vi "ZipUpCode.vi"() -> ()   [LabVIEW 2022 SP3]
uses:
  ViolinSubs/Mic/Mic_Global.vi
panel:
  out "error out":errorcluster
  out "Warnings":string
  out "Generated Zip File":path
  # "STEPS TO BUILD INSTALLERS\n\nZipUpCode first\n\nMac\n1. Build standalone - \n2. click on explore and compress the App folder\n2. drag it into the google drive\n\nPC \n0. grab zip file on the PC side - unzip\n1. open up Curtin1 in LabVIEW\n2. recompile and save all changes\n3. Build App\n4. build installer\n5. Zip up installer - and give it a name like ObieApp1_0b76\n6. copy that zip over to GoogleDrive:CurtinViolin:Code:PC"
  # "USE THE PC in the SHOP"
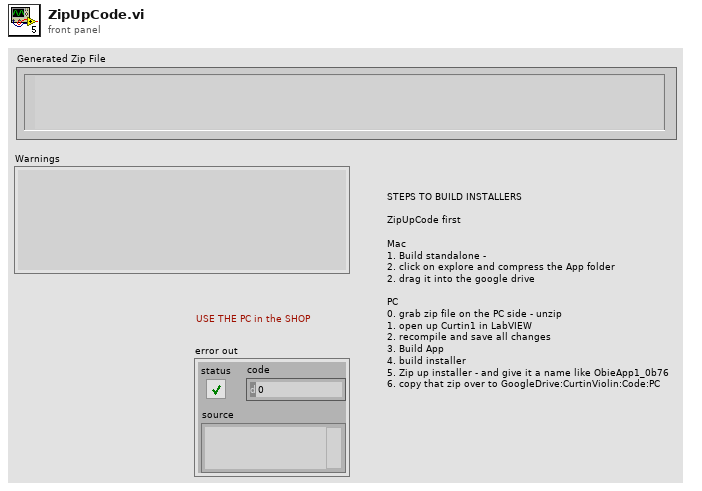
[diagram p1: front panel]
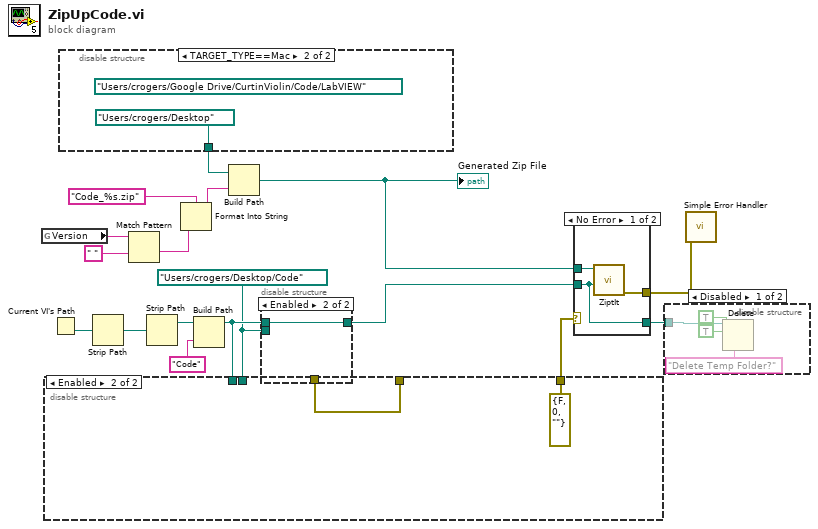
[diagram p0: block diagram]
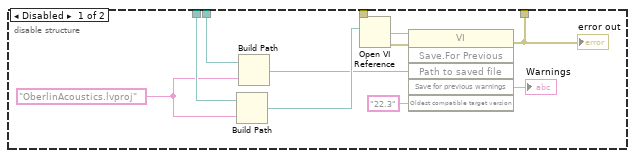
[diagram p3: hidden frame]
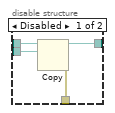
[diagram p4: hidden frame]
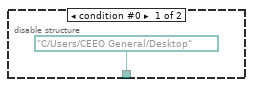
[diagram p6: hidden frame]
diagram:
  w1 = path "/Users/crogers/Desktop/Code"
  n1 = global read "Mic_Global.vi" "Version"() -> (w9:string)
  n2 = Current VI's Path() -> (path=w13:path)
  n3 = disable-structure shown="TARGET_TYPE==Mac" {
    disable-tunnel: [path "C:/Users/CEEO General/Desktop" ("default name") path "/Users/crogers/Desktop"] -> w18
    frame condition #0 {
    }
    frame condition #1 (active) {
      (unwired) path "/Users/crogers/Google Drive/CurtinViolin/Code/LabVIEW"
    }
  }
  n4 = Strip Path(path=w13) -> (stripped path=w12:path)  [unwired: 1 out]
  n5 = Match Pattern(string=w9, regular expression=" ") -> (after substring=w15:string)  [unwired: 1 in, 3 out]
  n6 = Strip Path(path=w12) -> (stripped path=w11:path)  [unwired: 1 out]
  n7 = Format Into String(format string="Code_%s.zip", w15) -> (resulting string=w14:string)  [unwired: 2 in, 1 out]
  n8 = Build Path(base path=w11, name or relative path="Code") -> (appended path=w2:path)
  n9 = Build Path(base path=w18, name or relative path=w14) -> (appended path=w8:path)
  "Generated Zip File" <- w8
  n10 = disable-structure shown="Enabled" {
    disable-tunnel: [w24 w25] -> w7
    disable-tunnel: w1 -> [w23 _]
    disable-tunnel: [w22 _] -> w6
    disable-tunnel: w2 -> [w21 w25]
    frame Disabled {
      n11 = Copy(10:w23, 11:w21) -> (0:w22:errorcluster, 3:w24:path)  [unwired: 3 in, 1 out]
    }
    frame Enabled {
    }
  }
  n12 = disable-structure shown="Enabled" {
    disable-tunnel: w6 -> [w32 _]
    disable-tunnel: [w30 errorcluster {"status"=FALSE, "code"=0, "source"=""} ("error out")] -> w5
    disable-tunnel: w2 -> [w29 _]
    disable-tunnel: w1 -> [w28 _]
    frame Disabled {
      w27 = "OberlinAcoustics.lvproj"
      n13 = Build Path(base path=w29, name or relative path=w27) -> (appended path=w35:path)
      n14 = Build Path(base path=w28, name or relative path=w27) -> (appended path=w26:path)
      n15 = Open VI Reference(vi path=w35, error in (no error)=w32) -> (vi reference=w36:refnum<vi>, error out=w31:errorcluster)  [unwired: 4 in]
      n16 = invoke class="VI" method="Save.For Previous"(reference=w36, error in=w31, "Path to saved file"=w26, "Oldest compatible target version"="22.3" ("Target Version")) -> (error out=w30:errorcluster, "Save for previous warnings"=→"Warnings":string)  [unwired: 2 in, 4 out]
      "error out" <- w30
    }
    frame Enabled {
    }
  }
  n17 = case shown="No Error" w5 {
    selector: w5 -> [_ w42]
    tunnel: w8 -> [w40 _]
    tunnel: w7 -> [w38 w41]
    tunnel: [w39 w42] -> w4
    tunnel: [w38 w41] -> w3
    frame No Error {
      n18 = call "ZiptIt.vi"("Folder to zip"=w38, "Zip file"=w40) -> ("error out"=w39:errorcluster)  [unwired: 8 in, 1 out]
    }
    frame Error {
    }
  }
  n19 = disable-structure shown="Disabled" {
    disable-tunnel: w3 -> [w46 _]
    frame Disabled {
      n20 = Delete(prompt (Delete)="Delete Temp Folder?", path (use dialog)=w46, entire hierarchy (F)=TRUE, confirm (F)=TRUE) -> ()  [unwired: 1 in, 3 out]
    }
    frame Enabled {
    }
  }
  n21 = call <vilib>:"Simple Error Handler.vi"("error in (no error)"=w4) -> ()  [unwired: 4 in, 5 out]
